vi "ADAM 5000 Relay Control.vi"(8 "Relay States IN":bool[](array[boolean]), 9 "State":bool=TRUE, 10 "Relay # (1=1st relay)":i32=1, 11 "Remote IP Address 2":string="192.168.10.200") -> (2 "Relay States OUT":bool[](array[boolean]))   [LabVIEW 2018]
uses:
  Adam Stuff/nimodbus121/71/vi.lib/NI Modbus.llb/MB Modbus Command.ctl
panel:
  in  "Modbus Command":T1={"Function Code"=15, "Starting Address"=17, "Quantity"=1, "Data"=[], "Discrete"=[]} {"Function Code" items=["Read Coils"=1, "Read Discrete Inputs"=2, "Read Holding Registers"=3, "Read Input Registers"=4, "Write Single Coil"=5, "Write Single Register"=6, "Read Exception Status"=7, "Write Multiple Coils"=15, "Write Multiple Registers"=16]}
  in  "Remote Port 2":u16=502
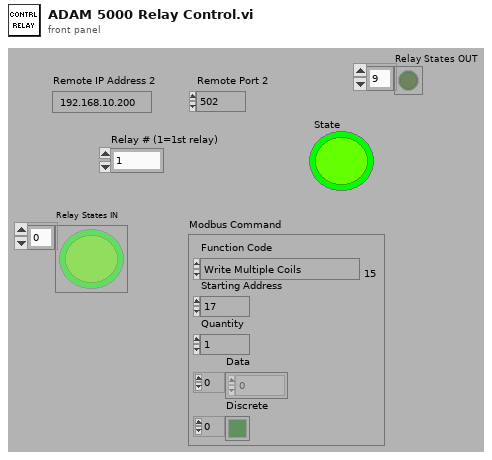
[diagram p1: front panel]
types:
  T1 = typedef "MB Modbus Command.ctl" = cluster{"Function Code":u8, "Starting Address":u16, "Quantity":u16, "Data":u16[], "Discrete":bool[]}
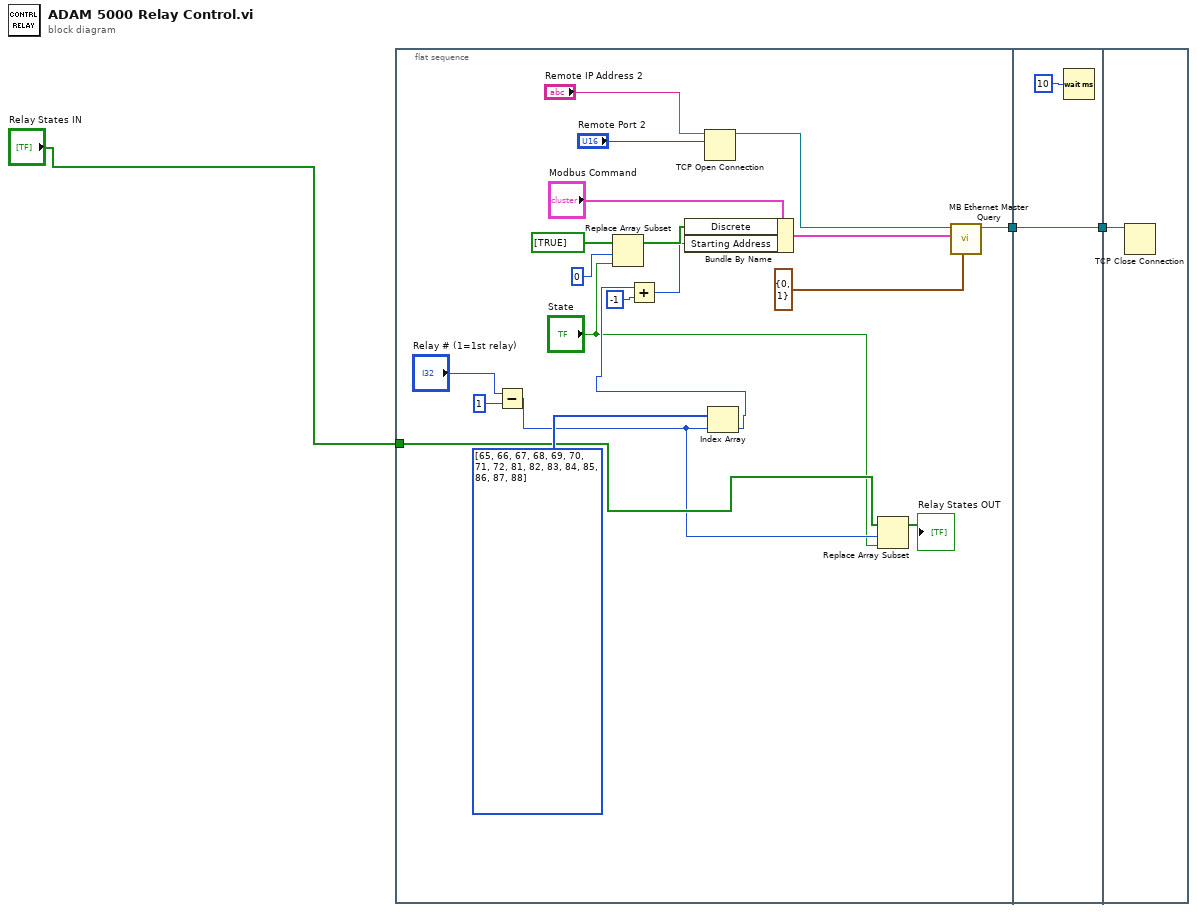
[diagram p0: block diagram]
diagram:
  n1 = flat-sequence {
    tunnel: [w12] -> w3
    tunnel: "Relay States IN" -> [w7]
    tunnel: w3 -> [w25]
    tunnel: [w25] -> w2
    tunnel: w2 -> [w26]
    frame #0 {
      n2 = Subtract(x="Relay # (1=1st relay)", y=1) -> (x-y=w6:i32)
      n3 = Replace Array Subset(array=bool[] [TRUE] ("Discrete"), new element="State", index=0) -> (w16:bool[])
      n4 = TCP Open Connection(address="Remote IP Address 2", remote port or service name="Remote Port 2") -> (connection ID=w21:refnum<k5>)  [unwired: 3 in, 1 out]
      n5 = Index Array(array=i32[] [65, 66, 67, 68, 69, 70, 71, 72, 81, 82, 83, 84, 85, 86, 87, 88], index=w6) -> (element=w8:i32)
      n6 = Add(x=w8, y=-1) -> (x+y=w14:i32)
      n7 = Bundle By Name(cluster="Modbus Command", "Discrete"=w16, "Starting Address"=w14) -> (w20:T1)
      n8 = Replace Array Subset(array=w7, new element="State", index=w6) -> (→"Relay States OUT":bool[])
      n9 = call "MB Ethernet Master Query.vi"("MBAP Header"=cluster{"Transaction ID":u16, "Unit ID":u8} {"Transaction ID"=0, "Unit ID"=1}, "Modbus Command"=w20, "TCP Connection Refnum in"=w21) -> ("TCP Connection Refnum (dup)"=w12:refnum<k5>)  [unwired: 4 in, 4 out]
    }
    frame #1 {
      n10 = Wait (ms)(milliseconds to wait=u32 10) -> ()  [unwired: 1 out]
    }
    frame #2 {
      n11 = TCP Close Connection(connection ID=w26) -> ()  [unwired: 2 in, 2 out]
    }
  }
